vi "Alphabetize Cluster Control Target.vi"() -> ()   [LabVIEW 2017, in "Tests.lvlib" / "Toolkit.lvlib"]
uses:
  Toolkit.lvlib
panel:
  out "Boolean":bool
  in  "String":string
  in  "Numeric":dbl
  in  "Data":T1
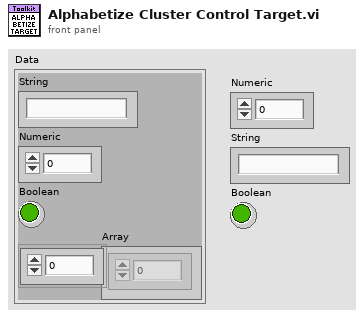
[diagram p1: front panel]
types:
  T1 = cluster{"String":string, "Numeric":dbl, "Boolean":bool, "Array":dbl[]}
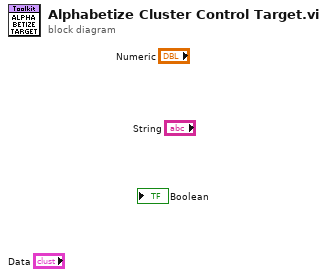
[diagram p0: block diagram]
diagram:
